vi "AD Set Output (Drivebase).vi"(2 "Control Mode":T1, 3 "Right":dbl, 4 "Left":dbl, 5 "Input cluster":cluster{"Left":string[], "Right":string[]}) -> ()   [LabVIEW 2019]
uses:
  <vilib>/Rock Robotics/WPI/ThirdParty/REV Robotics/SPARK MAX/Typedef/Spark MAX Control Type.ctl
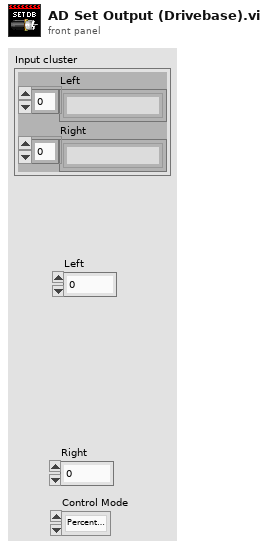
[diagram p1: front panel]
types:
  T1 = typedef "Spark MAX Control Type.ctl" = enum16{"Percent VBus", "Voltage", "Velocity", "Position", "Smart Motion", "Current", "Smart Velocity"}
  T2 = typedef "WPI_MotorControlDeviceRef.ctl" = cluster{"DeviceStatus":errorcluster, "Type":T3, "PWM":cluster{"PWM Channel":T4, "DeadBand":T5}, "CAN":cluster{"Device Number":u8, "SetOutput VI Ref":variant, "GetOutput VI Ref":variant, "Enable VI Ref":variant, "Disable VI Ref":variant, "Data":variant}, "Invert":bool, "DIO PWM":cluster{"PWM \"Enable\" Channel":T4, "DIOChannel":T6, "PWM Rate":dbl}}
  T3 = typedef "WPI_MotorControlType.ctl" = enum16{"PWM", "CAN", "DIO PWM"}
  T4 = typedef "FPGA_DIOPWMChannel.ctl" = enum8{"PWM 0", "PWM 1", "PWM 2", "PWM 3", "PWM 4", "PWM 5", "PWM 6", "PWM 7", "PWM 8", "PWM 9", "PWM MXP 0", "PWM MXP 1", "PWM MXP 2", "PWM MXP 3", "PWM MXP 4", "PWM MXP 5", "PWM MXP 6", "PWM MXP 7", "PWM MXP 8", "PWM MXP 9", "Invalid"}
  T5 = typedef "WPI_PWMDeadband.ctl" = cluster{"Name":string, "maxPositivePwm":i32, "minPositivePwm":i32, "centerPwm":i32, "maxNegativePwm":i32, "minNegativePwm":i32, "angularRange":u16}
  T6 = typedef "FPGA_DIOChannel.ctl" = enum8{"DIO 0", "DIO 1", "DIO 2", "DIO 3", "DIO 4", "DIO 5", "DIO 6", "DIO 7", "DIO 8", "DIO 9", "DIO MXP 0", "DIO MXP 1", "DIO MXP 2", "DIO MXP 3", "DIO MXP 4", "DIO MXP 5", "DIO MXP 6", "DIO MXP 7", "DIO MXP 8", "DIO MXP 9", "DIO MXP 10", "DIO MXP 11", "DIO MXP 12", "DIO MXP 13", "DIO MXP 14", "DIO MXP 15", "SPI Port CS1", "SPI Port CS2", "SPI Port CS3", "SPI Port MISO", "SPI Port MOSI", "Invalid"}
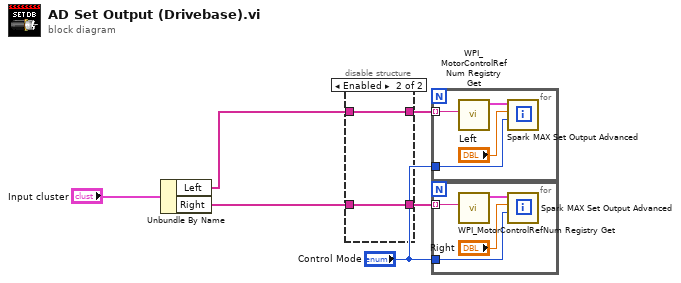
[diagram p0: block diagram]
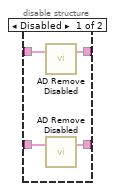
[diagram p2: hidden frame]
diagram:
  n1 = Unbundle By Name("Input cluster") -> ("Left"=w4:string[], "Right"=w2:string[])
  n2 = disable-structure shown="Enabled" {
    disable-tunnel: w4 -> [w10 w12]
    disable-tunnel: [w9 w12] -> w3
    disable-tunnel: w2 -> [w8 w11]
    disable-tunnel: [w7 w11] -> w1
    frame Disabled {
      n3 = call "AD Remove Disabled.vi"("Items In"=w10) -> ("Items Out"=w9:string[])  [unwired: 1 in, 1 out]
      n4 = call "AD Remove Disabled.vi"("Items In"=w8) -> ("Items Out"=w7:string[])  [unwired: 1 in, 1 out]
    }
    frame Enabled {
    }
  }
  n5 = for {
    tunnel: w3 -> [w16] mode=indexing
    tunnel: "Control Mode" -> [w14]
    n6 = call <vilib>:"WPI_MotorControlRefNum Registry Get.vi"("refnum name"=w16) -> ("MotorControlDevRef"=w15:T2)  [unwired: 9 in, 1 out]
    n7 = call <vilib>:"Spark MAX Set Output Advanced.vi"("Control Mode"=w14, "Setpoint"="Left", "MotorControlDevRef"=w15) -> ()  [unwired: 7 in, 2 out]
  }
  n8 = for {
    tunnel: w1 -> [w20] mode=indexing
    tunnel: "Control Mode" -> [w19]
    n9 = call <vilib>:"WPI_MotorControlRefNum Registry Get.vi"("refnum name"=w20) -> ("MotorControlDevRef"=w17:T2)  [unwired: 9 in, 1 out]
    n10 = call <vilib>:"Spark MAX Set Output Advanced.vi"("Control Mode"=w19, "Setpoint"="Right", "MotorControlDevRef"=w17) -> ()  [unwired: 7 in, 2 out]
  }
